vi "TestClient.vi"(8 "Error In":errorcluster, 10 "Data":variant, 11 "Queues":T1) -> ()   [LabVIEW 2017, in "Server.lvlib" / "Dialogs.lvlib"]
uses:
  Dialogs.lvlib
  Message Queue/CommReferences.ctl
  Message Queue/MessageCluster.ctl
  TestClientData.ctl
  ErrorLogger/ErrorLogger.lvlib
  <vilib>/httpClient/LabVIEWHTTPClient.lvlib
  Message Queue/Message Queue.lvlib
panel:
  out "HeartbeatBody":string
  out "HeartbeatHeader":string
  out "SRheader":string
  out "SRbody":string
  out "GetSR-Error":errorcluster
  in  "UpdateSRs":bool
  in  "Heartbeat Period (s)":dbl=10.0 format="%#_13g"
  in  "ClientName":string="TestClient"
  in  "Port":string="8001"
  in  "IP":string="localhost"
  out "HeartbeatError":errorcluster
  in  "Stop Button":bool
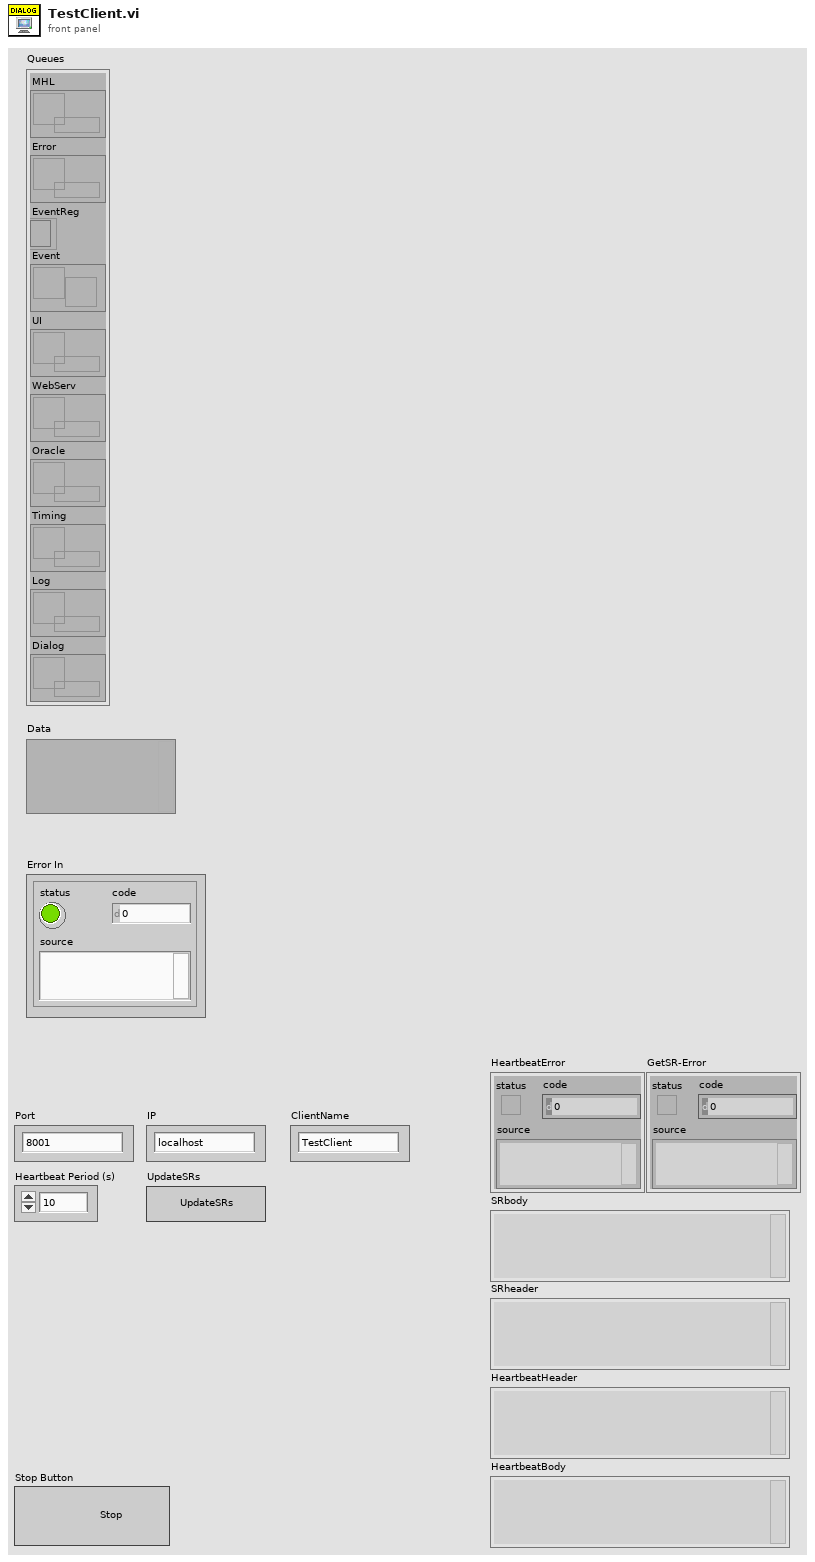
[diagram p1: front panel]
types:
  T1 = typedef "Server.lvlib/Message Queue.lvlib/CommReferences.ctl" = cluster{"MHL":refnum<queue>, "Error":refnum<queue>, "EventReg":refnum<event-registration>, "Event":refnum<user-event>, "UI":refnum<queue>, "WebServ":refnum<queue>, "Oracle":refnum<queue>, "Timing":refnum<queue>, "Log":refnum<queue>, "Dialog":refnum<queue>}
  T2 = typedef "Server.lvlib/Dialogs.lvlib/TestClientData.ctl" = cluster{"IP":string, "Port":string, "ClientName":string}
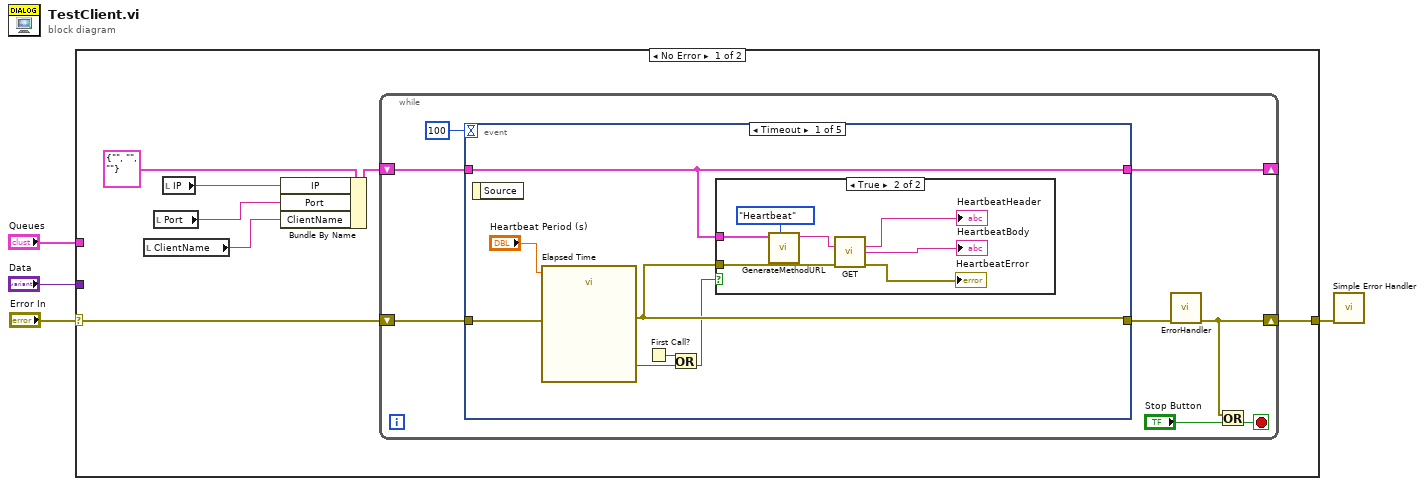
[diagram p0: block diagram]
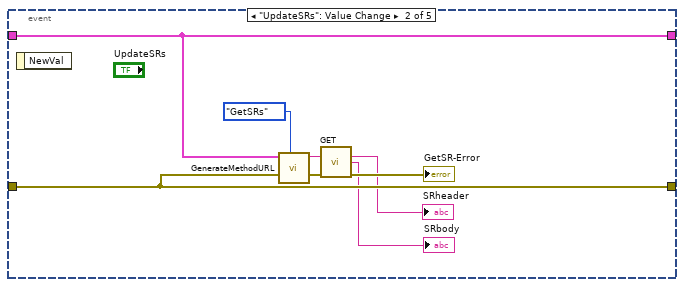
[diagram p3: hidden frame]
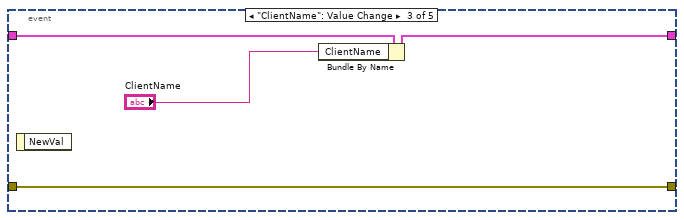
[diagram p4: hidden frame]
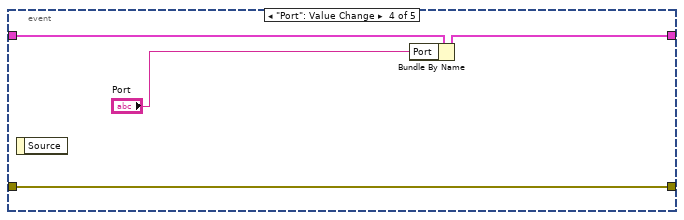
[diagram p5: hidden frame]
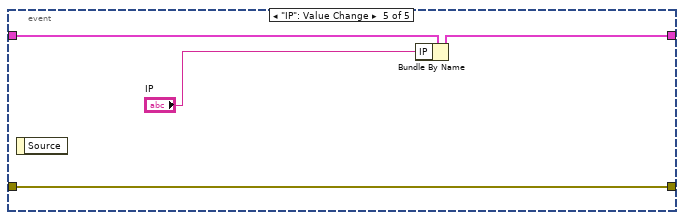
[diagram p6: hidden frame]
diagram:
  n1 = case shown="No Error" "Error In" {
    selector: "Error In" -> [w11 w53]
    tunnel: [w10 w53] -> w1
    tunnel: "Queues" -> [_ _]
    tunnel: "Data" -> [_ _]
    frame No Error {
      n2 = local read "ClientName"() -> (w5:string)
      n3 = local read "Port"() -> (w7:string)
      n4 = local read "IP"() -> (w6:string)
      n5 = Bundle By Name(cluster=T2 {"IP"="", "Port"="", "ClientName"=""}, "IP"=w6, "Port"=w7, "ClientName"=w5) -> (w8:T2)
      n6 = while {
        shift-right: [w16] -> w10
        shift-left: w11 -> [w19]
        shift-right: [w13] -> _
        shift-left: w8 -> [w12]
        stop <- w17 stop-if-true
        n7 = event shown="[0] Timeout" {
          selector: _ -> [_ _ _ _ _]
          dyn-events: _ -> [_ _ _ _ _]
          timeout: 100 -> [_ _ _ _ _]
          tunnel: w19 -> [w26 w37 w44 w47 w52]
          tunnel: [w25 w37 w44 w47 w52] -> w15
          tunnel: [w23 w40 w42 w46 w50] -> w13
          tunnel: w12 -> [w23 w40 w43 w48 w51]
          event Timeout {
            n8 = event-data() -> ()  [unwired: 1 in, 1 out]
            n9 = call "Elapsed Time"("Time Target (s)"="Heartbeat Period (s)", "error in (no error)"=w26) -> ("Time has Elapsed"=w24:bool, "error out"=w25:errorcluster)  [unwired: 10 in, 6 out]
            n10 = First Call?() -> (First Call?: T/F=w20:bool)
            n11 = Or(x=w20, y=w24) -> (x .or. y?=w21:bool)
            n12 = case shown="True" w21 {
              tunnel: w25 -> [_ w32]
              tunnel: w23 -> [_ w31]
              frame False {
              }
              frame True {
                n13 = call "GenerateMethodURL.vi"("Method"=enum16{"Heartbeat", "GetSRs"}."Heartbeat", "TestClientData"=w31) -> ("String"=w30:string)  [unwired: 9 in]
                n14 = call <vilib>:"GET.vi"("url"=w30, "error in (no error)"=w32) -> ("headers"=→"HeartbeatHeader":string, "body"=→"HeartbeatBody":string, "error out"=→"HeartbeatError":errorcluster)  [unwired: 10 in, 1 out]
              }
            }
          }
          event "UpdateSRs": Value Change {
            n15 = event-data() -> ()  [unwired: 1 in, 1 out]
            n16 = call "GenerateMethodURL.vi"("Method"=enum16{"Heartbeat", "GetSRs"}."GetSRs", "TestClientData"=w40) -> ("String"=w38:string)  [unwired: 9 in]
            n17 = call <vilib>:"GET.vi"("url"=w38, "error in (no error)"=w37) -> ("headers"=→"SRheader":string, "body"=→"SRbody":string, "error out"=→"GetSR-Error":errorcluster)  [unwired: 10 in, 1 out]
          }
          event "ClientName": Value Change {
            n18 = event-data() -> ()  [unwired: 1 in, 1 out]
            n19 = Bundle By Name(cluster=w43, "ClientName"="ClientName") -> (w42:T2)
          }
          event "Port": Value Change {
            n20 = event-data() -> ()  [unwired: 1 in, 1 out]
            n21 = Bundle By Name(cluster=w48, "Port"="Port") -> (w46:T2)
          }
          event "IP": Value Change {
            n22 = event-data() -> ()  [unwired: 1 in, 1 out]
            n23 = Bundle By Name(cluster=w51, "IP"="IP") -> (w50:T2)
          }
        }
        n24 = call "ErrorHandler.vi"("error in (no error)"=w15) -> ("error out"=w16:errorcluster)  [unwired: 10 in]
        n25 = Or(x=w16, y="Stop Button") -> (x .or. y?=w17:bool)
      }
    }
    frame Error {
    }
  }
  n26 = call <vilib>:"Simple Error Handler.vi"("error in (no error)"=w1) -> ()  [unwired: 4 in, 5 out]
